vi "set Main Texture Name.vi"(10 "Main Texture Name":string, 11 "Element in":refnum<class "Element.lvclass">) -> (3 "Element out":refnum<class "Element.lvclass">)   [LabVIEW 2021, in "Element.lvclass"]
uses:
  Element.lvclass
  Element.lvclass/Element.ctl
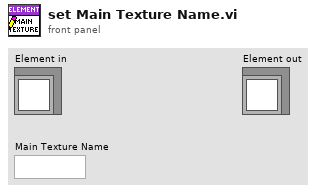
[diagram p1: front panel]
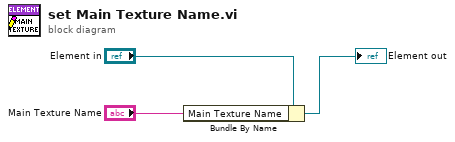
[diagram p0: block diagram]
diagram:
  n1 = Bundle By Name(cluster="Element in", "Main Texture Name"="Main Texture Name") -> (→"Element out":refnum<class "Element.lvclass">)
